vi "IMPORT Signals - File.vi"(0 "reference in":refnum<class "TDMS.lvclass">, 5 "error in (no error)":errorcluster, 7 "Grp/Sig Names":cluster{string, string}[](array[cluster]), 9 "TDMS Path - READ":path) -> (14 "reference out":refnum<class "TDMS.lvclass">, 19 "error out":errorcluster)   [LabVIEW 2022 SP3, in "TDMS.lvclass"]
uses:
  TDMS.lvclass
  API/GSwFormDSP_class/functions/Attribute List.ctl
  API/GSwFormDSP_class/GSwFormDSP.lvclass
  API/Generic Utilities_class/Generic Utilities.lvclass
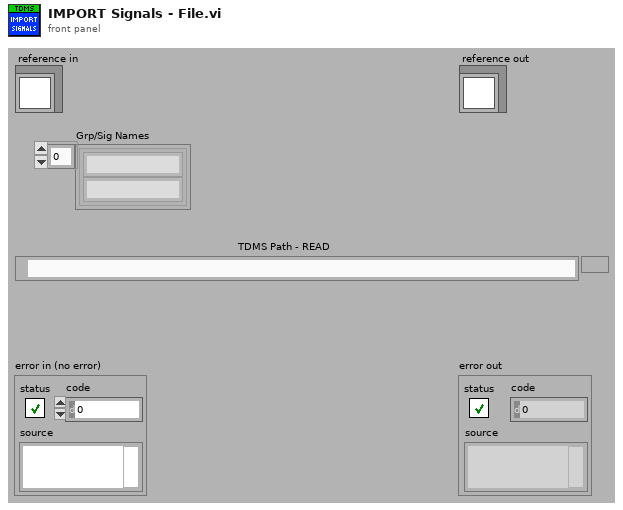
[diagram p1: front panel]
types:
  T1 = typedef "GSwFormDSP.lvclass/Attribute List.ctl" = string
  T2 = typedef "TDMS.lvclass/ObjectAttributesRef.ctl" = refnum<data-value>
  T3 = typedef "TDMS.lvclass/ObjectAttributes.ctl" = cluster{"Time Data":refnum<class "GSwFormDSP.lvclass">, "New Time Data Obj?":bool}
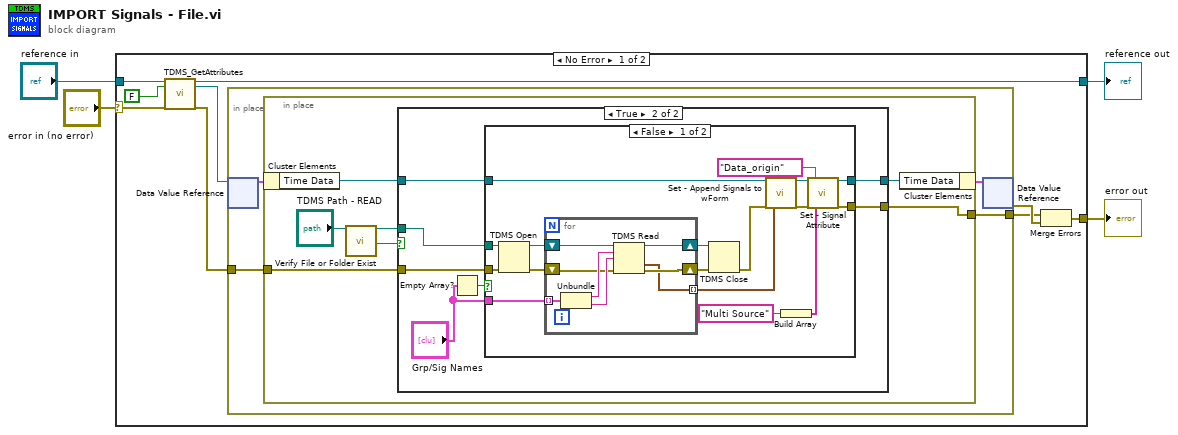
[diagram p0: block diagram]
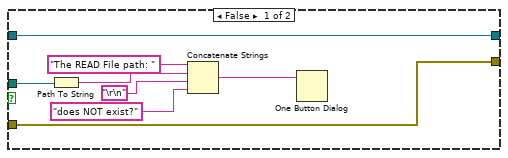
[diagram p2: hidden frame]
diagram:
  n1 = case shown="No Error" "error in (no error)" {
    selector: "error in (no error)" -> [w8 w68]
    tunnel: [w13 w68] -> w3
    tunnel: [w7 w67] -> w1
    tunnel: "reference in" -> [w10 w67]
    frame No Error {
      n2 = call "TDMS_GetAttributes.vi"("reference in"=w10, "return data? (T)"=FALSE, "error in (no error)"=w8) -> ("reference out"=w7:refnum<class "TDMS.lvclass">, "attributes ref"=w6:T2, "error out"=w5:errorcluster)  [unwired: 13 in, 1 out]
      n3 = in-place {
        in-place-border: [w14] -> w11
        in-place-border: w5 -> [w15]
        n4 = in-place-dvr #1(w6) -> (w16:T3)  [unwired: 1 out]
        n5 = in-place {
          in-place-border: w15 -> [w19]
          in-place-border: [w18] -> w14
          n6 = in-place-cluster #2(w16) -> ("Time Data"=w20:refnum<class "GSwFormDSP.lvclass">)
          n7 = call "Verify File or Folder Exist.vi"("path"="TDMS Path - READ") -> ("dup path"=w24:path, "file or folder exists?"=w23:bool)  [unwired: 16 in, 1 out]
          n8 = case shown="True" w23 {
            tunnel: w20 -> [w32 w39]
            tunnel: [w32 w37] -> w21
            tunnel: w24 -> [w30 w36]
            tunnel: w19 -> [w31 w35]
            tunnel: [w31 w38] -> w18
            frame False {
              n9 = Path To String(path=w30) -> (string=w28:string)
              n10 = Concatenate Strings("The READ File path: ", w28, "\r\n", "does NOT exist?") -> (w25:string)
              n11 = One Button Dialog(message=w25) -> ()  [unwired: 1 in, 1 out]
            }
            frame True {
              n12 = Empty Array?(array="Grp/Sig Names") -> (empty?=w33:bool)
              n13 = case shown="False" w33 {
                tunnel: w39 -> [w56 w66]
                tunnel: [w53 w65] -> w38
                tunnel: [w52 w66] -> w37
                tunnel: w36 -> [w46 _]
                tunnel: w35 -> [w45 w65]
                tunnel: "Grp/Sig Names" -> [w41 _]
                frame False {
                  n14 = TDMS Open(8:w45, 11:w46) -> (0:w51:errorcluster, 3:w50:refnum<k34>)  [unwired: 5 in]
                  n15 = for {
                    shift-right: [w63] -> w48
                    shift-left: w50 -> [w64]
                    shift-right: [w62] -> w49
                    shift-left: w51 -> [w58]
                    tunnel: w41 -> [w61] mode=indexing
                    tunnel: [w57] -> w40 mode=indexing
                    n16 = Unbundle(w61) -> (w60:string, w59:string)
                    n17 = TDMS Read(0:w64, 5:w60, 7:w59, 11:w58) -> (4:w63:refnum<k34>, 10:w57:waveform(dbl), 15:w62:errorcluster)  [unwired: 4 in, 3 out]
                  }
                  n18 = TDMS Close(8:w49, 11:w48) -> (0:w47:errorcluster)  [unwired: 1 out]
                  n19 = call "Set - Append Signals to wForm.vi"("reference in"=w56, "error in (no error)"=w47, "New Signals"=w40) -> ("reference out"=w55:refnum<class "GSwFormDSP.lvclass">, "error out"=w54:errorcluster)  [unwired: 15 in]
                  n20 = Build Array("Multi Source") -> (w44:string[])
                  n21 = call-dynamic "Set - Signal Attribute.vi"("reference in"=w55, "error in (no error)"=w54, "wForm Attributes"=T1 "Data_origin", "Attribute"=w44) -> ("reference in"=w52:refnum<class "GSwFormDSP.lvclass">, "error out"=w53:errorcluster)  [unwired: 14 in]
                }
                frame True {
                  # "NO Data to Import!"
                }
              }
            }
          }
          n22 = in-place-cluster #2("Time Data"=w21) -> (w17:T3)
        }
        n23 = in-place-dvr #1(w17) -> (w12:errorcluster)  [unwired: 1 out]
      }
      n24 = Merge Errors(w11, w12) -> (w13:errorcluster)
    }
    frame Error {
    }
  }
  "error out" <- w3
  "reference out" <- w1
